vi "Flywheel_Execute.vi"() -> ()   [LabVIEW 2020]
uses:
  Utility VIs/Basic_Motor_Modes.ctl
  Globals/Flywheel_Globals.vi
  Globals/Sensor_Values.vi
panel:
  out "Backspin_Error":dbl
  in  "Backspin_Acceptable_error":dbl=200.0
  out "Backspin_Error":cluster{dbl, dbl}(graph)
  in  "array":dbl[][](array[numeric])
  in  "Flywheel_MaxSpeed(RPM)":dbl=4900.0
  out "Error":cluster{dbl, dbl}(graph)
  out "Spun-Up":bool
  out "Error":dbl
  in  "Acceptable_error":dbl=200.0
  # "5500 max rpm on beta"
  # "Click here to set min"
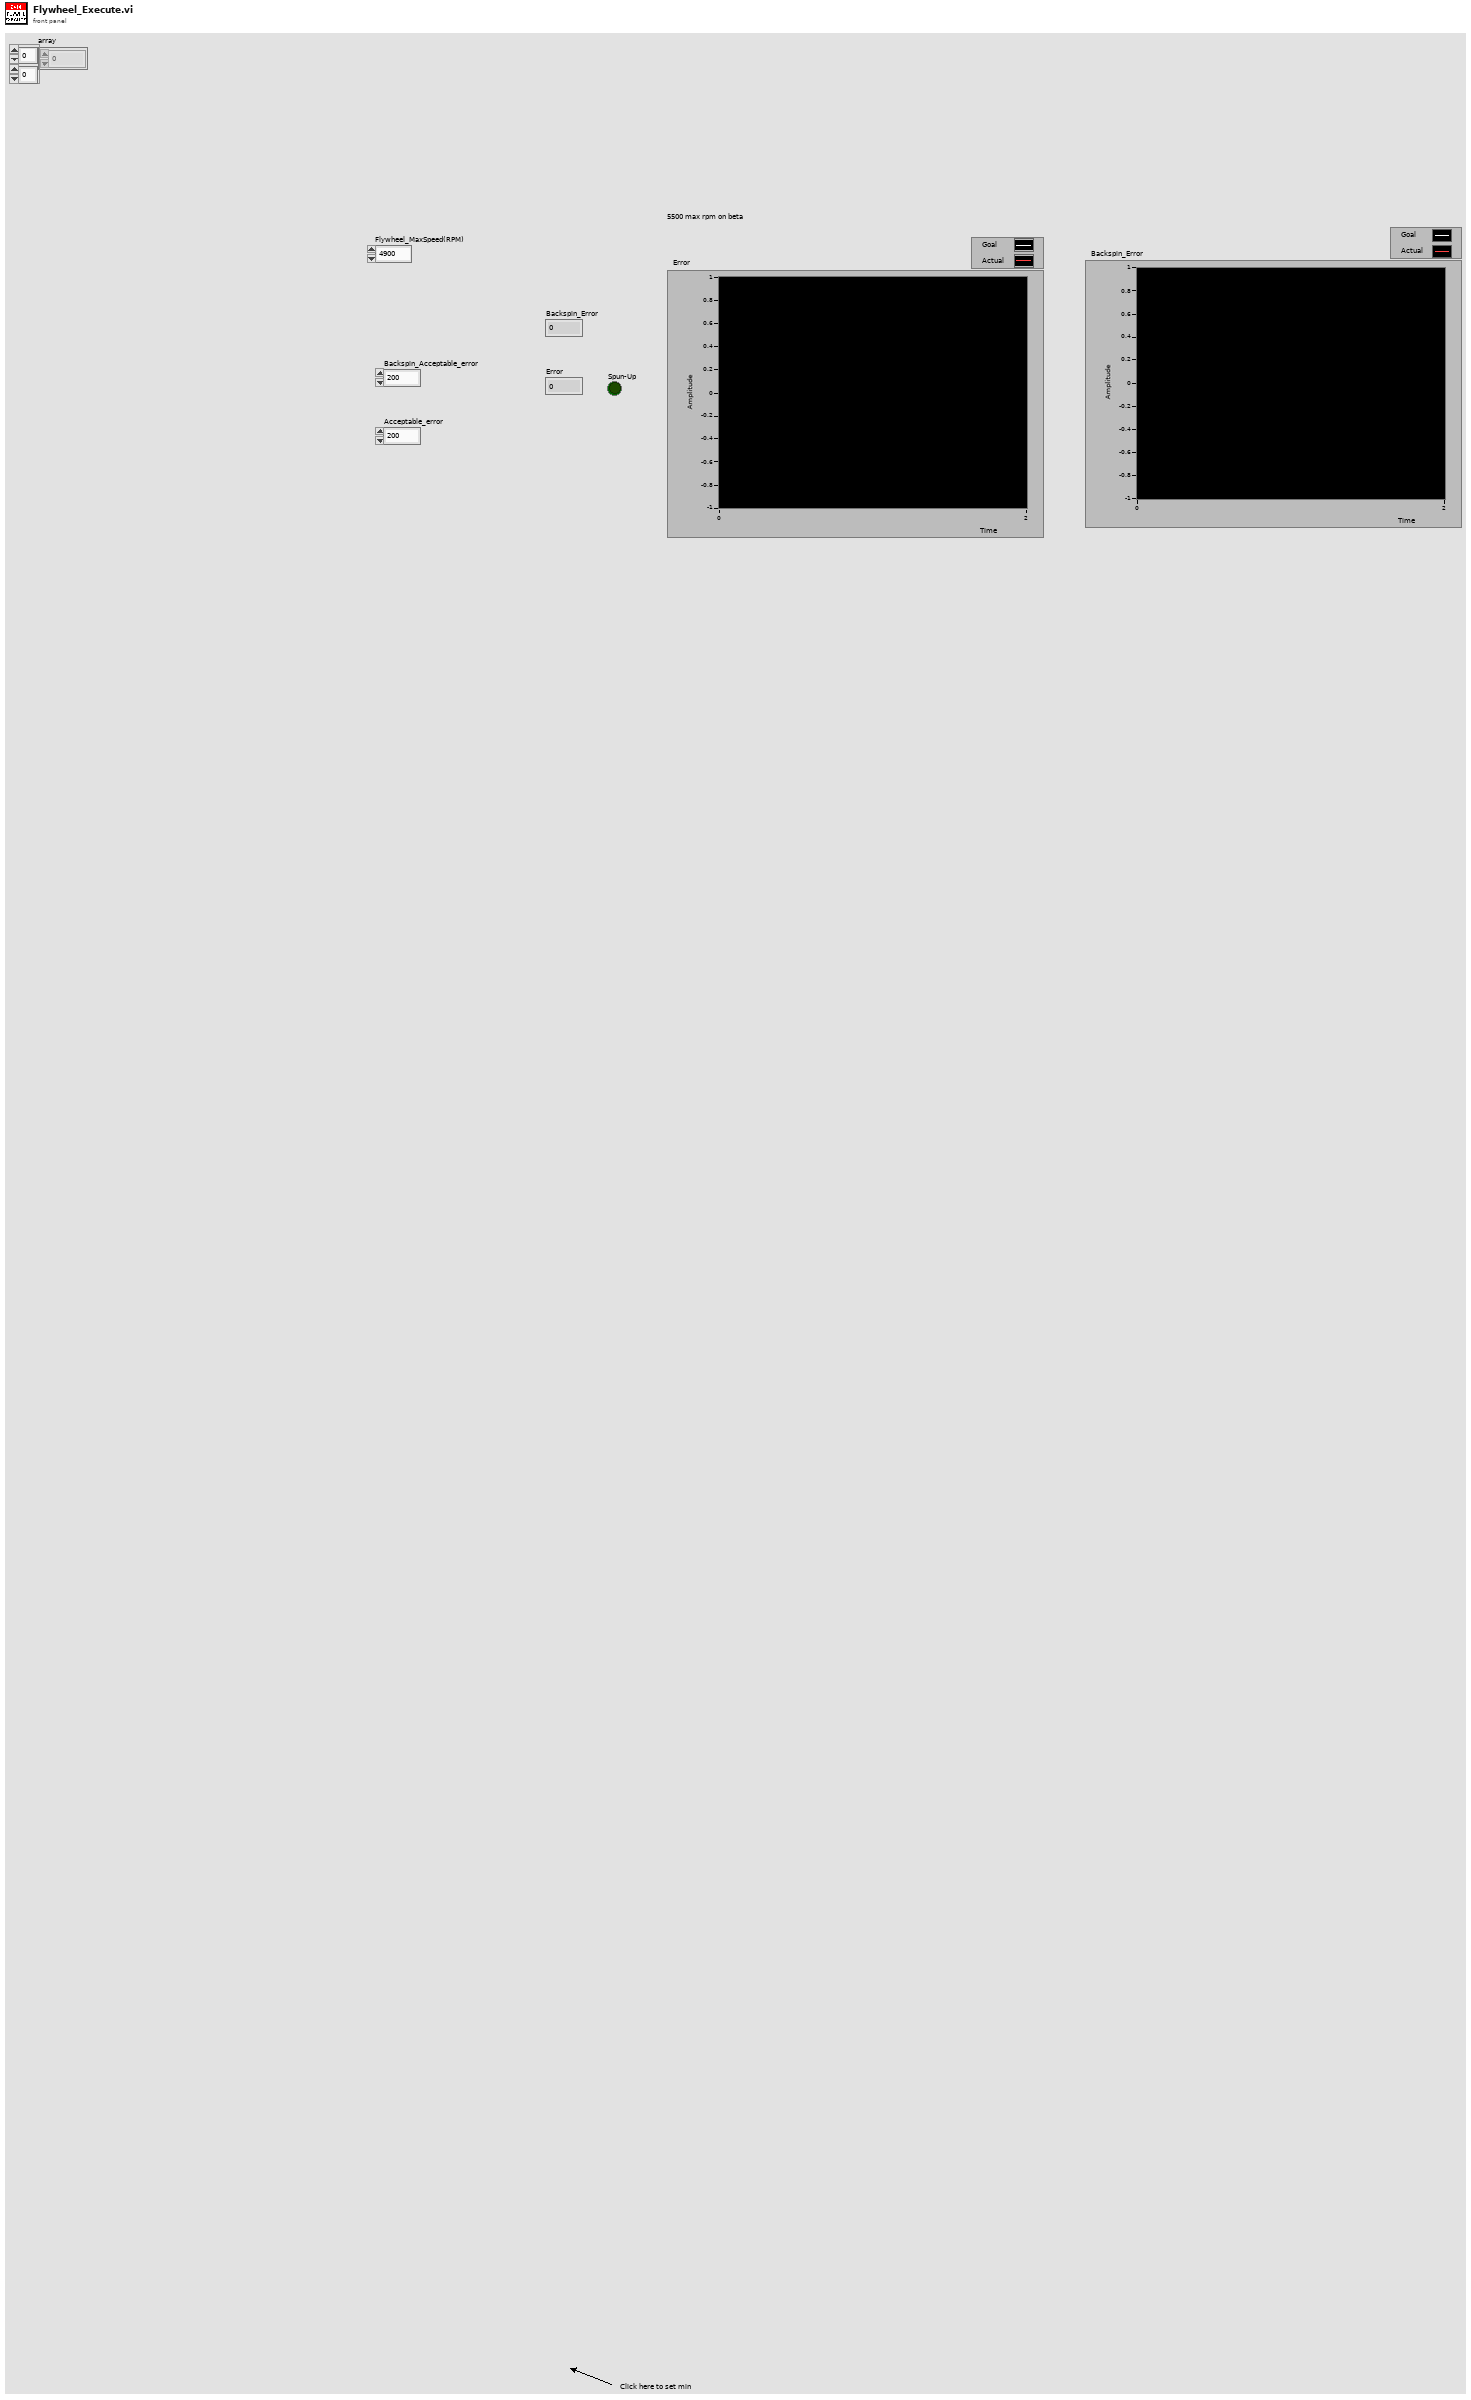
[diagram p1: front panel]
types:
  T1 = typedef "Basic_Motor_Modes.ctl" = enum16{"Percent_Voltage", "Speed_Control", "Position_Control", "Current"}
  T2 = typedef "Flywheel_Cluster.ctl" = cluster{"Flywheel_Throttle":dbl, "Flywheel_Control_State":T3, "Parameter_1":dbl, "Parameter_2":dbl, "Auto_Notifier":refnum<notifier>, "Step":dbl, "Flywheel_Velocity_Goal":dbl, "Flywheel_On ":bool}
  T3 = typedef "Flywheel_States.ctl" = enum16{"No-Op", "Percent_Voltage", "Speed_Control", "Speed_Control_Manual", "Command_SpinUp", "Command_SpinUpAuto"}
  T4 = cluster{"Flywheel_Velocity_Goal":dbl, "Backspin_Flywheel_Velocity(RPM)":dbl}
  T5 = cluster{"Flywheel_Velocity_Goal":dbl, "Flywheel_Velocity(RPM)":dbl}
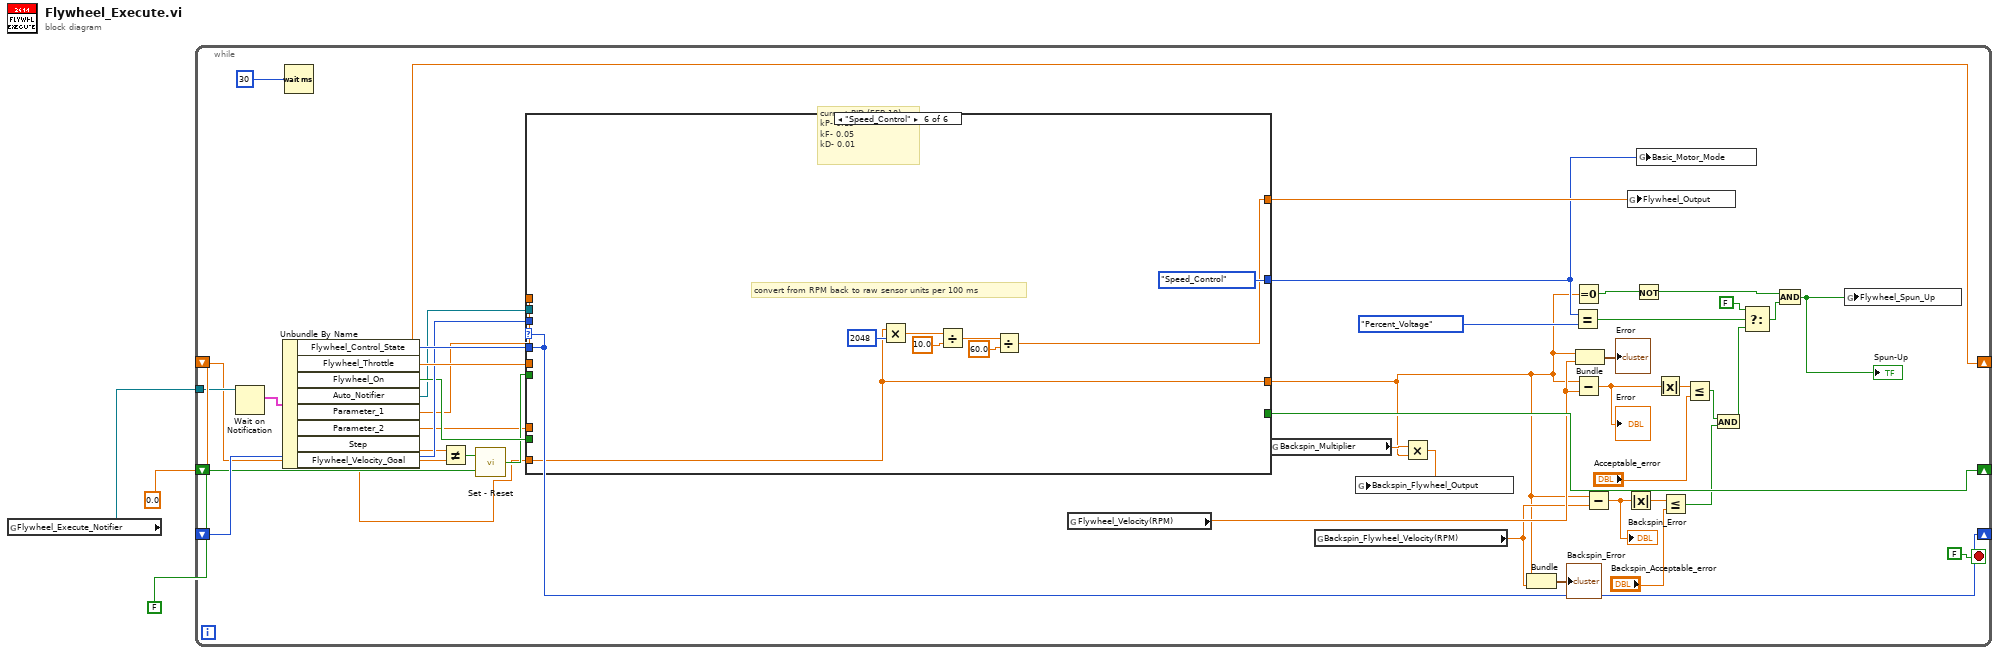
[diagram p0: block diagram]
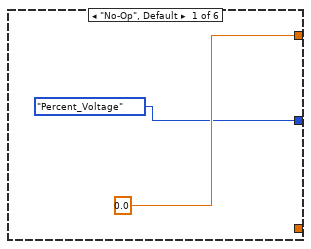
[diagram p2: hidden frame]
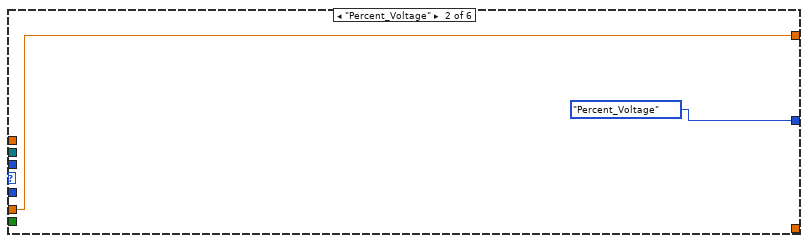
[diagram p3: hidden frame]
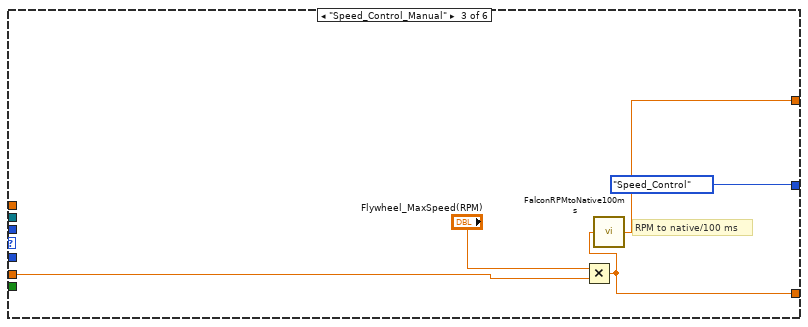
[diagram p4: hidden frame]
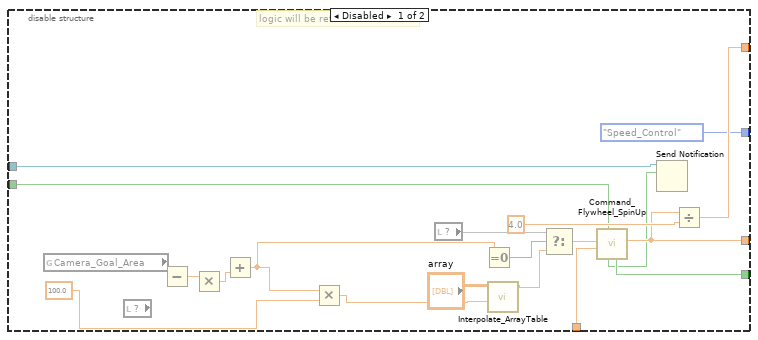
[diagram p6: hidden frame]
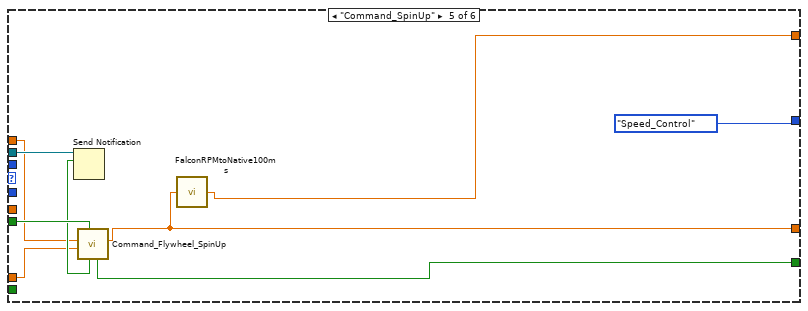
[diagram p7: hidden frame]
diagram:
  # "current PID (FEB 18)\nkP- 0.15\nkF- 0.05\nkD- 0.01"
  n1 = global read "Flywheel_Globals.vi" "Flywheel_Execute_Notifier"() -> (w3:refnum<notifier>)
  n2 = while {
    tunnel: w3 -> [w45]
    shift-right: [w41] -> _
    shift-left: _ -> [w40]
    shift-right: [w23] -> _
    shift-left: 0.0 ("Step") -> [w22]
    shift-right: [w28] -> _
    shift-left: FALSE ("Reint") -> [w29]
    stop <- FALSE stop-if-true
    n3 = Wait on Notification(notifier=w45) -> (notification=w44:T2)  [unwired: 3 in, 3 out]
    n4 = Unbundle By Name(w44) -> ("Flywheel_Control_State"=w41:T3, "Flywheel_Throttle"=w43:dbl, "Flywheel_On"=w33:bool, "Auto_Notifier"=w27:refnum<notifier>, "Parameter_1"=w26:dbl, "Parameter_2"=w25:dbl, "Step"=w23:dbl, "Flywheel_Velocity_Goal"=w17:dbl)
    n5 = Wait (ms)(milliseconds to wait=u32 30) -> ()  [unwired: 1 out]
    n6 = Not Equal?(x=w23, y=w22) -> (x != y?=w24:bool)
    n7 = call "Set - Reset.vi"("Reset"=w29, "Set"=w24) -> ("Output"=w30:bool)
    n8 = case shown="\"Speed_Control\"" w41 {
      tunnel: [0.0 ("Flywheel_Throttle") w50 w51 w62 w84 w93] -> w21
      tunnel: w43 -> [_ w50 w55 _ _ _]
      tunnel: w41 -> [_ _ _ _ _ _]
      tunnel: w40 -> [_ _ _ _ _ _]
      tunnel: [_ _ w52 w61 w83 w92] -> w4
      tunnel: w33 -> [_ _ _ _ _ _]
      tunnel: w30 -> [_ _ _ w59 w91 _]
      tunnel: [_ _ _ w58 w90 _] -> w28
      tunnel: w27 -> [_ _ _ w57 w89 _]
      tunnel: w26 -> [_ _ _ _ w87 _]
      tunnel: w25 -> [_ _ _ w60 w86 _]
      tunnel: [Basic_Motor_Modes."Percent_Voltage" ("Motor_Mode") Basic_Motor_Modes."Percent_Voltage" ("Motor_Mode") Basic_Motor_Modes."Speed_Control" ("Motor_Mode") w56 Basic_Motor_Modes."Speed_Control" ("Motor_Mode") Basic_Motor_Modes."Speed_Control" ("Motor_Mode")] -> w19
      tunnel: w17 -> [_ _ _ _ _ w92]
      frame "No-Op", Default {
      }
      frame "Percent_Voltage" {
      }
      frame "Speed_Control_Manual" {
        # "RPM to native/100 ms"
        n9 = Multiply(x="Flywheel_MaxSpeed(RPM)", y=w55) -> (x*y=w52:dbl)
        n10 = call "FalconRPMtoNative100ms.vi"("RPM"=w52) -> ("raw sensor units / 100 ms"=w51:dbl)  [unwired: 4 in]
      }
      frame "Command_SpinUpAuto" {
        n11 = disable-structure shown="Enabled" {
          disable-tunnel: [w81 _] -> w62
          disable-tunnel: [w76 _] -> w61
          disable-tunnel: w60 -> [w75 _]
          disable-tunnel: w59 -> [w74 _]
          disable-tunnel: [w73 _] -> w58
          disable-tunnel: w57 -> [w72 _]
          disable-tunnel: [Basic_Motor_Modes."Speed_Control" ("Motor_Mode") _] -> w56
          frame Disabled {
            # "logic will be retuned with m14"
            n12 = global read "Sensor_Values.vi" "Camera_Goal_Area"() -> (w67)
            n13 = local read item#-1() -> ()  [unwired: 1 out]
            n14 = Subtract() -> (x-y=w66:dbl)  [unwired: 2 in]
            n15 = Multiply(x=w66) -> (x*y=w65:dbl)  [unwired: 1 in]
            n16 = Add(y=w65) -> (x+y=w68:dbl)  [unwired: 1 in]
            n17 = Multiply(x=w68, y=100.0) -> (x*y=w69:dbl)
            n18 = local read item#-1() -> (w78)
            n19 = Equal To 0?(x=w68) -> (x = 0?=w79:bool)
            n20 = call "Interpolate_ArrayTable.vi"("Desired_Distance"=w69, "array"="array") -> ("RPM"=w70:dbl)  [unwired: 9 in]
            n21 = Select(t=w78, s=w79, f=w70) -> (s? t:f=w77:dbl)
            n22 = call "Command_Flywheel_SpinUp.vi"("Startup"=w74, "Timeout"=w75, "Speed"=w77) -> ("Flywheel_Output"=w76:dbl, "Reint"=w73:bool, "Completed"=w71:bool)  [unwired: 6 in]
            n23 = Send Notification(notification=w71, notifier=w72) -> ()  [unwired: 1 in, 2 out]
            n24 = Divide(x=w76, y=4.0) -> (x/y=w81:dbl)
          }
          frame Enabled {
          }
        }
      }
      frame "Command_SpinUp" {
        n25 = call "Command_Flywheel_SpinUp.vi"("Startup"=w91, "Timeout"=w86, "Speed"=w87) -> ("Flywheel_Output"=w83:dbl, "Reint"=w90:bool, "Completed"=w88:bool)  [unwired: 6 in]
        n26 = Send Notification(notification=w88, notifier=w89) -> ()  [unwired: 1 in, 2 out]
        n27 = call "FalconRPMtoNative100ms.vi"("RPM"=w83) -> ("raw sensor units / 100 ms"=w84:dbl)  [unwired: 4 in]
      }
      frame "Speed_Control" {
        # "convert from RPM back to raw sensor units per 100 ms"
        n28 = Multiply(x=w92, y=2048) -> (x*y=w97:dbl)
        n29 = Divide(x=w97, y=10.0) -> (x/y=w95:dbl)
        n30 = Divide(x=w95, y=60.0) -> (x/y=w93:dbl)
      }
    }
    n31 = global read "Sensor_Values.vi" "Flywheel_Velocity(RPM)"() -> (w18:dbl)
    n32 = global read "Flywheel_Globals.vi" "Backspin_Multiplier"() -> (w6:dbl)
    n33 = global read "Sensor_Values.vi" "Backspin_Flywheel_Velocity(RPM)"() -> (w12:dbl)
    n34 = Multiply(x=w6, y=w4) -> (x*y=w5:dbl)
    n35 = global write "Flywheel_Globals.vi" "Backspin_Flywheel_Output"(w5) -> ()
    n36 = Bundle("Flywheel_Velocity_Goal"=w4, "Backspin_Flywheel_Velocity(RPM)"=w12) -> (→"Backspin_Error":T4)  [unwired: 1 in]
    n37 = Equal?(x=w19, y=Basic_Motor_Modes."Percent_Voltage" ("Motor_Mode")) -> (x = y?=w37:bool)
    n38 = Equal To 0?(x=w4) -> (x = 0?=w16:bool)
    n39 = Subtract(x=w4, y=w18) -> (x-y=w35:dbl)
    "Error" <- w35
    n40 = Bundle("Flywheel_Velocity_Goal"=w4, "Flywheel_Velocity(RPM)"=w18) -> (→"Error":T5)  [unwired: 1 in]
    n41 = Subtract(x=w4, y=w12) -> (x-y=w11:dbl)
    "Backspin_Error" <- w11
    n42 = Absolute Value(x=w11) -> (abs(x)=w10:dbl)
    n43 = global write "Flywheel_Globals.vi" "Flywheel_Output"(w21) -> ()
    n44 = Not(x=w16) -> (.not. x?=w15:bool)
    n45 = global write "Flywheel_Globals.vi" "Basic_Motor_Mode"(w19) -> ()
    n46 = Absolute Value(x=w35) -> (abs(x)=w39:dbl)
    n47 = Less Or Equal?(x=w10, y="Backspin_Acceptable_error") -> (x <= y?=w7:bool)
    n48 = Less Or Equal?(x=w39, y="Acceptable_error") -> (x <= y?=w8:bool)
    n49 = And(x=w8, y=w7) -> (x .and. y?=w9:bool)
    n50 = Select(t=FALSE, s=w37, f=w9) -> (s? t:f=w32:bool)
    n51 = And(x=w15, y=w32) -> (x .and. y?=w31:bool)
    "Spun-Up" <- w31
    n52 = global write "Flywheel_Globals.vi" "Flywheel_Spun_Up"(w31) -> ()
  }
